vi "ELVIS III v1.0 Unreserve AI IRQ.vi"(8 "error in (no error)":errorcluster, 10 "IO IRQ Channels Enum":T1) -> (0 "error out":errorcluster)   [LabVIEW 2021]
uses:
  <vilib>/myRIO/Common/Instrument Driver Framework/myRIO v1.0/IRQ/typedefs/IO IRQ Channels Enum.ctl
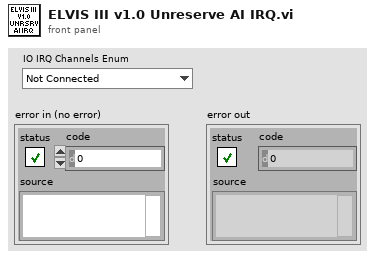
[diagram p1: front panel]
types:
  T1 = typedef "IO IRQ Channels Enum.ctl" = enum16{"Not Connected", "A/AI0 (Interrupt)", "A/AI1 (Interrupt)", "A/DIO0 (Interrupt)", "A/DIO1 (Interrupt)", "A/DIO2 (Interrupt)", "A/DIO3 (Interrupt)", "Button0 (Interrupt)", "B/AI0 (Interrupt)", "B/AI1 (Interrupt)", "B/DIO0 (Interrupt)", "B/DIO1 (Interrupt)", "B/DIO2 (Interrupt)", "B/DIO3 (Interrupt)"}
  T2 = typedef "ELVIS III v1.0 Channel Reservation List.ctl" = T3[]
  T3 = typedef "ELVIS III v1.0 Channel Reservation Info.ctl" = cluster{"Channel Name":string, "Connector":T4, "MutexIDs":u32[]}
  T4 = typedef "ELVIS III v1.0 Connector List.ctl" = enum32{"None", "ConnectorA", "ConnectorB"}
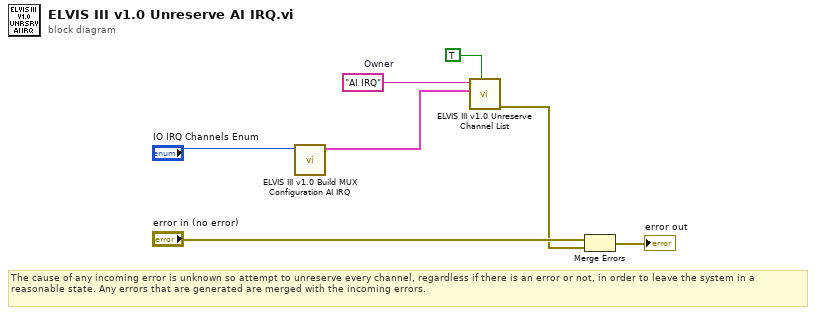
[diagram p0: block diagram]
diagram:
  w4 = "AI IRQ"  # Owner
  # "The cause of any incoming error is unknown so attempt to unreserve every channel, regardless if there is an error or not, in order to leave the system in a reasonable state. Any errors that are generated are merged with the incoming errors."
  n1 = call <vilib>:"ELVIS III v1.0 Build MUX Configuration AI IRQ.vi"("IO IRQ Channels Enum"="IO IRQ Channels Enum") -> ("Channel Reservation Info"=w5:T2)  [unwired: 10 in]
  n2 = call <vilib>:"ELVIS III v1.0 Unreserve Channel List.vi"("Allow multiple opens?"=TRUE, "Channel Reservation List"=w5, "Owner"=w4) -> ("error out"=w3:errorcluster)  [unwired: 8 in]
  n3 = Merge Errors("error in (no error)", w3) -> (→"error out":errorcluster)
